vi "HyperTerminal Table.vi"(9 "Page Selector":T1=enum."User Page", 11 "read buffer":string) -> (3 "HyperTerminal Table":picture[][](array[picture]))   [LabVIEW 2018]
doc: "This VI is ment to replicate the Hyperterminal screen used to communicate and configure a Serial COMs device that expects a VT100 terminal. It provides the ability to configure the device through labview, and thus eliminating the need to stop LabVIEW in the middle of a Test in order to make configuration changes.\n\nIt takes in the raw data stream from the device, and converts it into a 2D array table.\nThe data comes in using ANSI Escape Sequence code. This code can be intepreted by a hyperterminal emulator (i.e. PuTTY), but it is not comparable with LabVIEW. \n\nThis VI is reponsible for presenting the data as a reasily readable table, while removing empty, or irelevant data."
uses:
  Page Selector.ctl
  <vilib>/regexp/Match Regular Expression.xnode
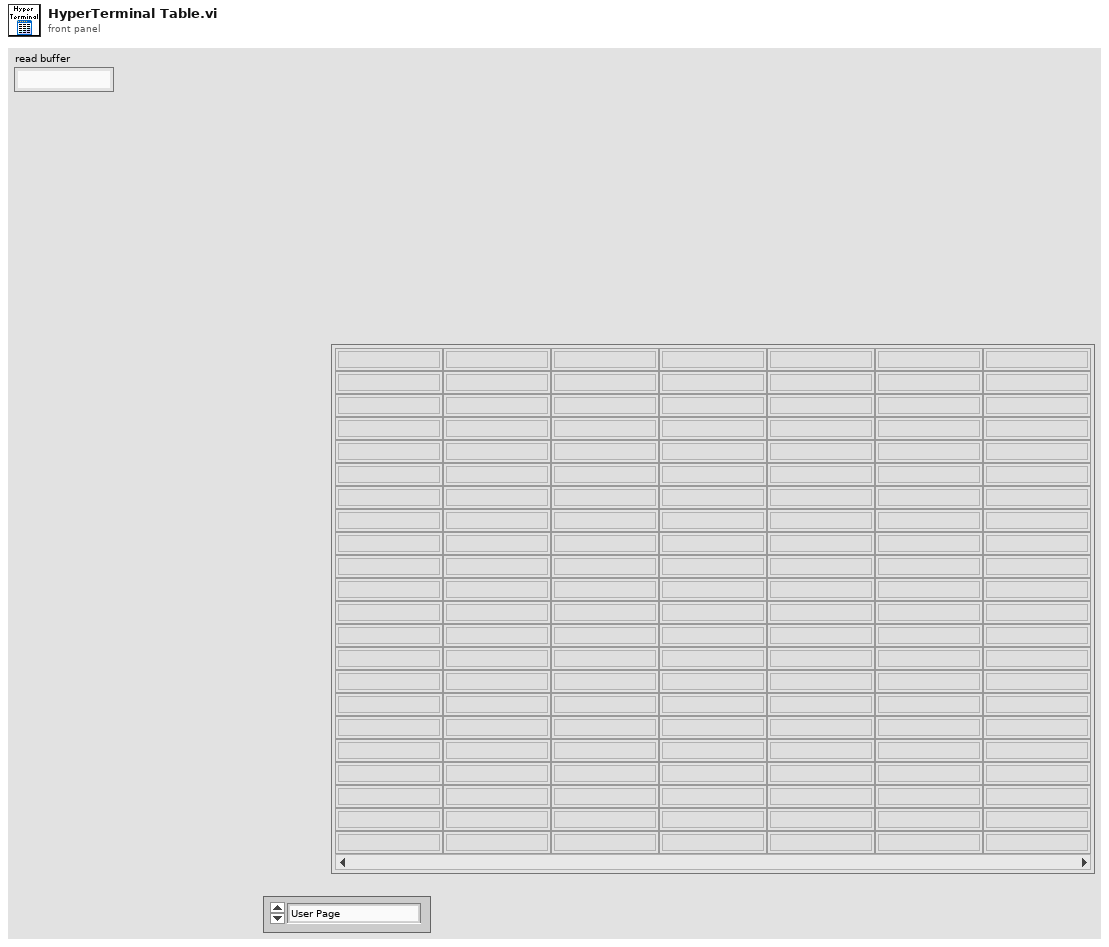
[diagram p1: front panel]
types:
  T1 = typedef "Page Selector.ctl" = enum16{"TLC Page", "User Page", "FBI Page", "HBI Page", "OSR Page", "Status Page", "Comms Page", "Diagnostic Page"}
  T2 = cluster{"left":i16, "top":i16, "right":i16, "bottom":i16}
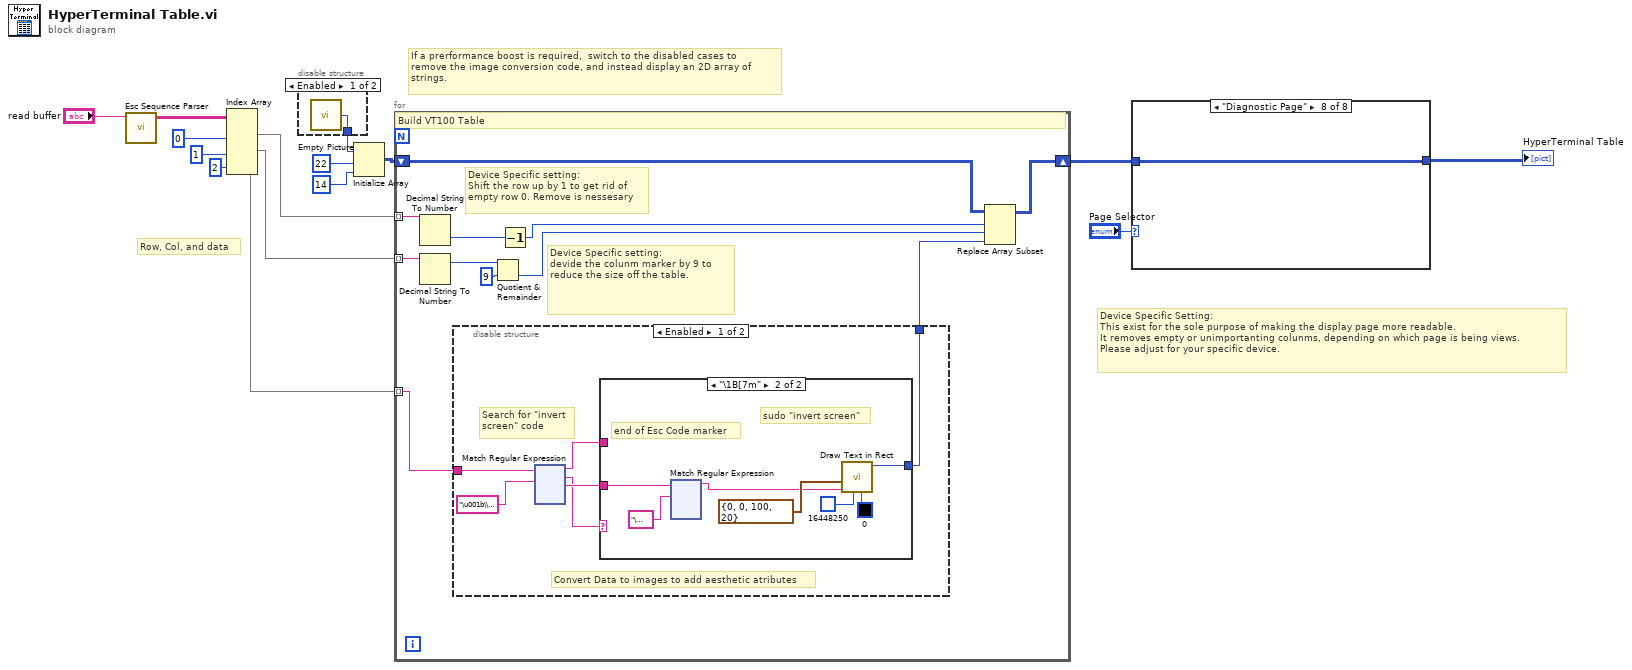
[diagram p0: block diagram]
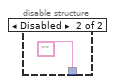
[diagram p2: hidden frame]
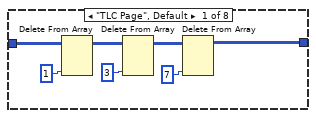
[diagram p3: hidden frame]
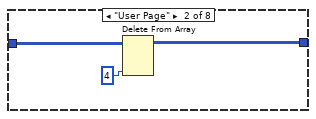
[diagram p4: hidden frame]
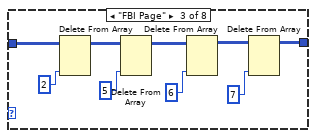
[diagram p5: hidden frame]
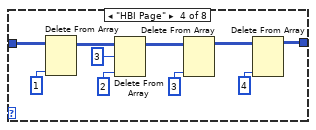
[diagram p6: hidden frame]
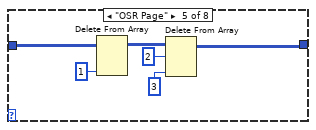
[diagram p7: hidden frame]
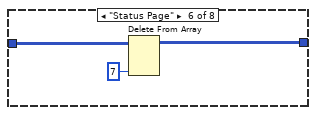
[diagram p8: hidden frame]
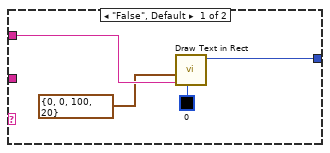
[diagram p10: hidden frame]
diagram:
  # "If a prerformance boost is required,  switch to the disabled cases to\nremove the image conversion code, and instead display an 2D array of\nstrings."
  # "Device Specific Setting:\nThis exist for the sole purpose of making the display page more readable.\nIt removes empty or unimportanting colunms, depending on which page is being views.\nPlease adjust for your specific device."
  # "Row, Col, and data"
  n1 = call "Esc Sequence Parser.vi"("read buffer"="read buffer") -> ("Array"=w14:string[][])  [unwired: 10 in]
  n2 = Index Array(array=w14, index (col) #1=0 ("index (row)"), index (col) #2=1 ("index (col)"), index (col) #3=2 ("index (col)")) -> (element #1=w10:string[], element #2=w9:string[], element #3=w8:string[])  [unwired: 3 in]
  n3 = disable-structure shown="Enabled" {
    disable-tunnel: [w16 ""] -> w4
    frame Enabled {
      n4 = call "Empty Picture"() -> ("empty picture"=w16:picture)
    }
    frame Disabled {
    }
  }
  n5 = Initialize Array(w4, 22 ("dimension size"), 14 ("dimension size")) -> (w7:picture[][])
  n6 = for {
    shift-right: [w26] -> w2
    shift-left: w7 -> [w20]
    tunnel: w10 -> [w28] mode=indexing
    tunnel: w9 -> [w27] mode=indexing
    tunnel: w8 -> [w19] mode=indexing
    # "Device Specific setting: \nShift the row up by 1 to get rid of\nempty row 0. Remove is nessesary"
    # "Device Specific setting: \ndevide the colunm marker by 9 to reduce the size off the table."
    # "Build VT100 Table"
    n7 = Decimal String To Number(string=w28) -> (number=w22:i32)  [unwired: 2 in, 1 out]
    n8 = Decimal String To Number(string=w27) -> (number=w25:i32)  [unwired: 2 in, 1 out]
    n9 = disable-structure shown="Enabled" {
      disable-tunnel: w19 -> [w30 w274]
      disable-tunnel: [w29 w274] -> w18
      frame Enabled {
        # "Convert Data to images to add aesthetic atributes"
        # "Search for \"invert\nscreen\" code"
        n10 = xnode "Match Regular Expression"("input string"=w30, "regular expression"="\u001b\\[7m" ("string")) -> ("before match"=w32:string, "whole match"=w31:string, "after match"=w33:string)  [unwired: 4 in, 2 out]
        n11 = case shown="\"\\1B[7m\"" w31 {
          tunnel: w33 -> [_ w159]
          tunnel: w32 -> [w152 _]
          tunnel: [w149 w154] -> w29
          frame "False", Default {
            n12 = call <vilib>:"Draw Text in Rect.vi"("text color(black)"=u32 0, "text"=w152, "rect"=T2 {"left"=0, "top"=0, "right"=100, "bottom"=20}) -> ("new picture"=w149:picture)  [unwired: 8 in]
          }
          frame "\u001b[7m" {
            # "sudo \"invert screen\""
            # "end of Esc Code marker"
            n13 = xnode "Match Regular Expression"("input string"=w159, "regular expression"="\u001b\\[" ("string")) -> ("before match"=w155:string)  [unwired: 4 in, 4 out]
            n14 = call <vilib>:"Draw Text in Rect.vi"("BG color(transparent)"=u32 0, "text color(black)"=u32 16448250, "text"=w155, "rect"=T2 {"left"=0, "top"=0, "right"=100, "bottom"=20}) -> ("new picture"=w154:picture)  [unwired: 7 in]
          }
        }
      }
      frame Disabled {
      }
    }
    n15 = Quotient & Remainder(x=w25, y=9) -> (floor(x/y)=w23:i32)  [unwired: 1 out]
    n16 = Decrement(x=w22) -> (x-1=w21:i32)
    n17 = Replace Array Subset(array=w20, new element=w18, index (row)=w21, index (col)=w23) -> (w26:picture[][])
  }
  n18 = case shown="\"Diagnostic Page\"" "Page Selector" {
    tunnel: w2 -> [w281 w284 w292 w302 w306 w311 w313 w314]
    tunnel: [w275 w282 w285 w295 w305 w310 w313 w314] -> w1
    frame "TLC Page", Default {
      n19 = Delete From Array(array=w281, index (col)=1 ("disabled index (col)")) -> (array with subset deleted=w278:picture[][])  [unwired: 2 in, 1 out]
      n20 = Delete From Array(array=w278, index (col)=3 ("disabled index (col)")) -> (array with subset deleted=w276:picture[][])  [unwired: 2 in, 1 out]
      n21 = Delete From Array(array=w276, index (col)=7 ("disabled index (col)")) -> (array with subset deleted=w275:picture[][])  [unwired: 2 in, 1 out]
    }
    frame "User Page" {
      n22 = Delete From Array(array=w284, index (col)=4 ("disabled index (col)")) -> (array with subset deleted=w282:picture[][])  [unwired: 2 in, 1 out]
    }
    frame "FBI Page" {
      n23 = Delete From Array(array=w292, index (col)=2 ("disabled index (col)")) -> (array with subset deleted=w290:picture[][])  [unwired: 2 in, 1 out]
      n24 = Delete From Array(array=w290, index (col)=5 ("disabled index (col)")) -> (array with subset deleted=w288:picture[][])  [unwired: 2 in, 1 out]
      n25 = Delete From Array(array=w288, index (col)=6 ("disabled index (col)")) -> (array with subset deleted=w286:picture[][])  [unwired: 2 in, 1 out]
      n26 = Delete From Array(array=w286, index (col)=7 ("disabled index (col)")) -> (array with subset deleted=w285:picture[][])  [unwired: 2 in, 1 out]
    }
    frame "HBI Page" {
      n27 = Delete From Array(array=w302, index (col)=1 ("disabled index (col)")) -> (array with subset deleted=w301:picture[][])  [unwired: 2 in, 1 out]
      n28 = Delete From Array(array=w301, length=3, index (col)=2 ("disabled index (col)")) -> (array with subset deleted=w300:picture[][])  [unwired: 1 in, 1 out]
      n29 = Delete From Array(array=w300, index (col)=3 ("disabled index (col)")) -> (array with subset deleted=w297:picture[][])  [unwired: 2 in, 1 out]
      n30 = Delete From Array(array=w297, index (col)=4 ("disabled index (col)")) -> (array with subset deleted=w295:picture[][])  [unwired: 2 in, 1 out]
    }
    frame "OSR Page" {
      n31 = Delete From Array(array=w306, index (col)=1 ("disabled index (col)")) -> (array with subset deleted=w309:picture[][])  [unwired: 2 in, 1 out]
      n32 = Delete From Array(array=w309, length=2, index (col)=3 ("disabled index (col)")) -> (array with subset deleted=w305:picture[][])  [unwired: 1 in, 1 out]
    }
    frame "Status Page" {
      n33 = Delete From Array(array=w311, index (col)=7 ("disabled index (col)")) -> (array with subset deleted=w310:picture[][])  [unwired: 2 in, 1 out]
    }
    frame "Comms Page" {
    }
    frame "Diagnostic Page" {
    }
  }
  "HyperTerminal Table" <- w1
